vi "Secured Setting.vi"(8 "error in (no error)":errorcluster, 9 "Secured Setting (82: Locked)":u16(ring)=82 items=["Locked"=82, "Unlocked"=64], 10 "Node (3)":u8=3 caption="Node" min=3 max=128 step=1, 11 "VISA resource name":refnum<visa-resource-name>) -> (0 "error out":errorcluster, 3 "VISA resource name out":refnum<visa-resource-name>)   [LabVIEW 2024, in "Bronkhorst FLOW-BUS.lvlib"]
doc: "Writes 82 or 64 to the init/reset parameter to disable or enable writing to secured parameters."
uses:
  Bronkhorst FLOW-BUS.lvlib
  Private/FLOW-BUS RW.ctl
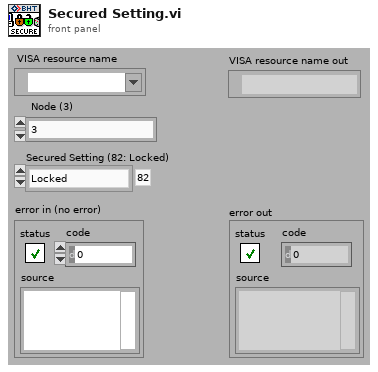
[diagram p1: front panel]
types:
  T1 = typedef "Bronkhorst FLOW-BUS.lvlib/FLOW-BUS RW.ctl" = cluster{"Node Address (3)":u8, "Communication Command":enum16{"Status message", "Send parameter with destination address and 00 response", "Send parameter with destination address", "Request parameter"}, "Process (0)":u16, "Parameter (0)":u16, "Data Type (0: Character)":enum16{"Character", "Integer", "Float or Long", "String"}, "Data for Char or Int (0)":u32, "Data for Float or Long (0)":sgl, "Data for String":string, "Length of Requested String (0)":u8}
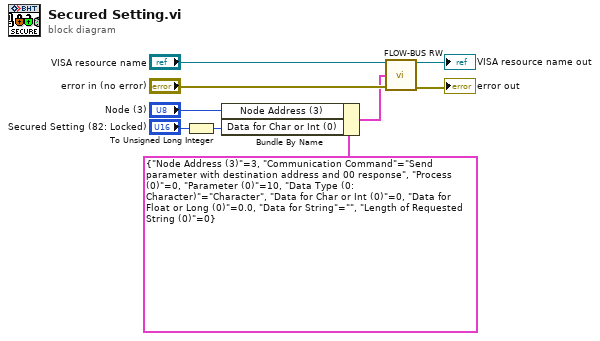
[diagram p0: block diagram]
diagram:
  n1 = To Unsigned Long Integer(number="Secured Setting (82: Locked)") -> (unsigned 32bit integer=w4:u32)
  n2 = Bundle By Name(cluster=T1 {"Node Address (3)"=3, "Communication Command"=enum."Send parameter with destination address and 00 response", "Process (0)"=0, "Parameter (0)"=10, "Data Type (0: Character)"=enum."Character", "Data for Char or Int (0)"=0, "Data for Float or Long (0)"=0.0, "Data for String"="", "Length of Requested String (0)"=0} ("FLOW-BUS Command Settings"), "Node Address (3)"="Node (3)", "Data for Char or Int (0)"=w4) -> (w2:T1)
  n3 = call "FLOW-BUS RW.vi"("VISA resource name"="VISA resource name", "FLOW-BUS Command Settings"=w2, "error in (no error)"="error in (no error)") -> ("VISA resource name out"=→"VISA resource name out":refnum<visa-resource-name>, "error out"=→"error out":errorcluster)  [unwired: 8 in, 3 out]
